vi "LoadClass.vi"(0 "reference in":refnum<class "DAQ_Base.lvclass">, 1 "ClassName":string="NI_DAQ", 5 "error in (no error)":errorcluster) -> (14 "reference out":refnum<class "DAQ_Base.lvclass">, 19 "error out":errorcluster)   [LabVIEW 2020, in "DAQ_Base.lvclass"]
uses:
  DAQ_Base.lvclass
  <vilib>/addons/_AddQ/G#Object/G#Object.lvclass
panel:
  out "LibRootPath":path
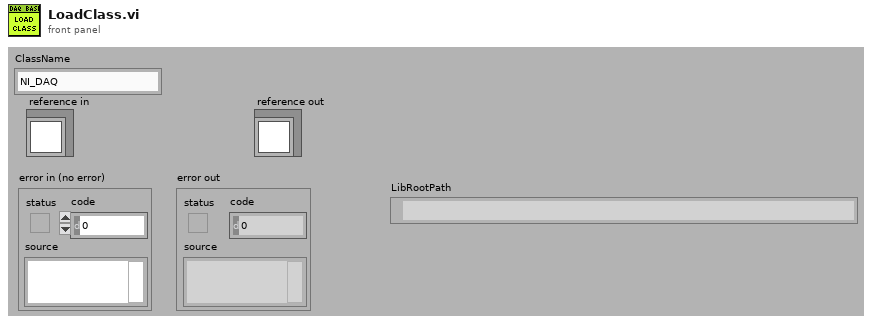
[diagram p1: front panel]
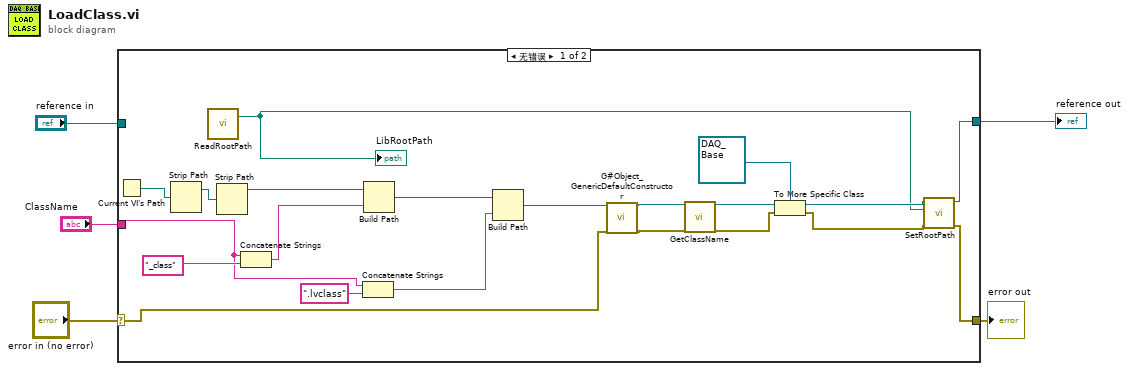
[diagram p0: block diagram]
diagram:
  n1 = case shown="无错误" "error in (no error)" {
    selector: "error in (no error)" -> [w12 w28]
    tunnel: [w8 w28] -> w4
    tunnel: "reference in" -> [_ w27]
    tunnel: "ClassName" -> [w13 _]
    tunnel: [w9 w27] -> w1
    frame No Error {
      n2 = Current VI's Path() -> (path=w24:path)
      n3 = Strip Path(path=w24) -> (stripped path=w25:path)  [unwired: 1 out]
      n4 = call "ReadRootPath.vi"() -> ("Root path"=w6:path)  [unwired: 19 in]
      "LibRootPath" <- w6
      n5 = Strip Path(path=w25) -> (stripped path=w26:path)  [unwired: 1 out]
      n6 = Concatenate Strings(w13, "_class" ("name or relative path")) -> (w20:string)
      n7 = Concatenate Strings "Concatenate Strings"(w13, ".lvclass" ("string")) -> (w17:string)
      n8 = Build Path(base path=w26, name or relative path=w20) -> (appended path=w16:path)
      n9 = Build Path(base path=w16, name or relative path=w17) -> (appended path=w21:path)
      n10 = call <vilib>:"G#Object_GenericDefaultConstructor.vi"("class path"=w21, "error in (no error)"=w12) -> ("reference out"=w22:refnum<class "G#Object.lvclass">, "error out"=w23:errorcluster)  [unwired: 15 in, 1 out]
      n11 = call-dynamic "GetClassName.vi"("reference in"=w22, "error in (no error)"=w23) -> ("reference out"=w15:refnum<class "G#Object.lvclass">, "error out"=w14:errorcluster)  [unwired: 13 in, 3 out]
      n12 = To More Specific Class(target class=refnum<class "DAQ_Base.lvclass"> refnum ("Base"), reference=w15, error in=w14) -> (specific class reference=w11:refnum<class "DAQ_Base.lvclass">, error out=w10:errorcluster)
      n13 = call-dynamic "SetRootPath.vi"("error in (no error)"=w10, "RootPath"=w6, "reference in"=w11) -> ("error out"=w8:errorcluster, "reference out"=w9:refnum<class "DAQ_Base.lvclass">)  [unwired: 7 in]
    }
    frame Error {
    }
  }
  "error out" <- w4
  "reference out" <- w1
